vi "test Invalid Event References Leaking.vi"(8 "error in":errorcluster) -> (0 "error out":errorcluster)   [LabVIEW 2020, in "ase.test.lvlib"]
uses:
  ase.test.lvlib
  ase/ase/ase.lvclass/ase.ctl
  ase/ase/Trim Whitespace.vi
  ase/ase/Merge Call Library Errors.vi
  ase/ase/Check Shared Library Version.vi
  ase/ase/Start Call.vi/a70fc713-9ee9-4497-bede-7e71c94245f2.vi
  ase/ase/Error Invalid ASE Handle.vi
  ase/ase/Error Internal Library Implementation Error.vi
  <vilib>/Utility/file.llb/Application Directory.vi
  ase/ase/Wait on Call.vi
  <vilib>/addons/_JKI Toolkits/Caraya/classes/Assert/Assert Equal Value_Variant.vi
  ase/ase/ase.lvclass
  <vilib>/addons/_JKI Toolkits/Caraya/classes/Assert/Assert.lvclass
  <vilib>/addons/_JKI Toolkits/Caraya/classes/Test/Test.lvclass
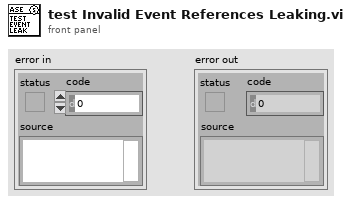
[diagram p1: front panel]
types:
  T1 = typedef "ase.lvlib/ase.lvclass/Event References.ctl" = cluster{"Standard Output":refnum<user-event>, "Standard Error":refnum<user-event>, "Did Exit":refnum<user-event>}
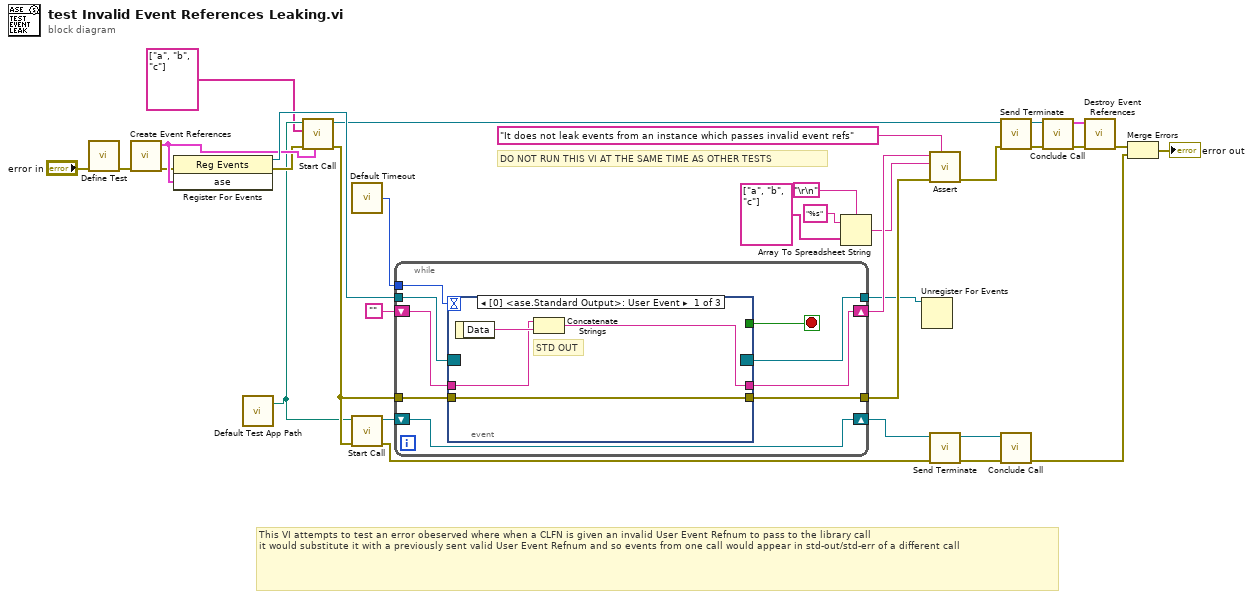
[diagram p0: block diagram]
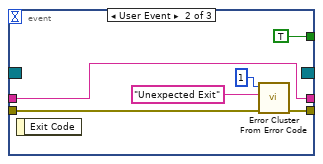
[diagram p2: hidden frame]
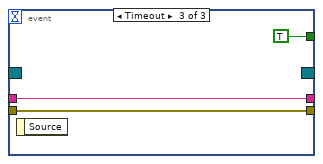
[diagram p3: hidden frame]
diagram:
  # "This VI attempts to test an error obeserved where when a CLFN is given an invalid User Event Refnum to pass to the library call\nit would substitute it with a previously sent valid User Event Refnum and so events from one call would appear in std-out/std-err of a different call"
  # "DO NOT RUN THIS VI AT THE SAME TIME AS OTHER TESTS"
  n1 = call <vilib>:"Define Test.vi"("error in (no error)"="error in") -> ("error out"=w27:errorcluster)  [unwired: 9 in, 1 out]
  n2 = call "Create Event References.vi"("error in"=w27) -> ("error out"=w25:errorcluster, "ase"=w28:T1)  [unwired: 9 in]
  n3 = register-events(error in=w25, w28) -> (reference out=w30:refnum<event-registration>, error out=w26:errorcluster)  [unwired: 1 in]
  n4 = call "Default Test App Path.vi"() -> ("Exe Path With Extention"=w3:path)  [unwired: 2 in, 1 out]
  n5 = call "Start Call.vi"("Event References"=w28, "error in"=w26, "Arguments (Default: Empty)"=string[] ["a", "b", "c"] ("Arguments"), "Executable Path"=w3) -> ("error out"=w15:errorcluster, "New ASE Handle"=w17:refnum<class "ase.lvclass">)  [unwired: 6 in]
  n6 = call "Default Timeout.vi"() -> ("Default Timeout"=w31:i32)
  n7 = call "Start Call.vi"("error in"=w15, "Executable Path"=w3) -> ("error out"=w14:errorcluster, "New ASE Handle"=w12:refnum<class "ase.lvclass">)  [unwired: 8 in]
  n8 = while {
    tunnel: w30 -> [w41]
    tunnel: [w40] -> w1
    shift-right: [w37] -> w21
    shift-left: "" ("Empty String Constant") -> [w38]
    tunnel: w31 -> [w36]
    tunnel: [w42] -> w20
    tunnel: w15 -> [w35]
    shift-right: [w34] -> w13
    shift-left: w12 -> [w34]
    stop <- w39 stop-if-true
    n9 = event shown="[0] <ase.Standard Output>: User Event" {
      selector: w41 -> [_ _ _]
      dyn-events: [_ _ _] -> w40
      timeout: w36 -> [_ _ _]
      tunnel: [w43 w50 w53] -> w42
      tunnel: [_ TRUE TRUE] -> w39
      tunnel: w38 -> [w45 w52 w54]
      tunnel: [w44 w52 w54] -> w37
      tunnel: w35 -> [w43 w47 w53]
      event User Event {
        # "STD OUT"
        n10 = event-data() -> ("Data"=w46:string)  [unwired: 1 in]
        n11 = Concatenate Strings(w45, w46) -> (w44:string)
      }
      event User Event {
        n12 = event-data() -> ()  [unwired: 1 in, 1 out]
        n13 = call <vilib>:"Error Cluster From Error Code.vi"("error in (no error)"=w47, "error message (\"\")"="Unexpected Exit" ("error message (\"\")"), "error code (0)"=1) -> ("error out"=w50:errorcluster)  [unwired: 6 in]
      }
      event Timeout {
        n14 = event-data() -> ()  [unwired: 1 in, 1 out]
      }
    }
  }
  n15 = Array To Spreadsheet String(delimiter (Tab)="\r\n", array=string[] ["a", "b", "c"] ("Arguments"), 3:"%s" ("format string")) -> (spreadsheet string=w4:string)
  n16 = Unregister For Events(event registration refnum=w1) -> ()  [unwired: 1 in, 1 out]
  n17 = call-poly <vilib>:"Assert.vi"("Label"="It does not leak events from an instance which passes invalid event refs", "error in (no error)"=w20, "Y"=w4, "X"=w21) -> ("error out"=w24:errorcluster)  [unwired: 6 in, 1 out]
  n18 = call "Send Terminate.vi"("error in"=w14, "ASE Handle"=w13) -> ("error out"=w10:errorcluster, "ASE Handle Duplicate"=w11:refnum<class "ase.lvclass">)  [unwired: 7 in, 1 out]
  n19 = call "Send Terminate.vi"("error in"=w24, "ASE Handle"=w17) -> ("error out"=w18:errorcluster, "ASE Handle Duplicate"=w16:refnum<class "ase.lvclass">)  [unwired: 7 in, 1 out]
  n20 = call "Conclude Call.vi"("error in"=w10, "ASE Handle"=w11) -> ("error out"=w8:errorcluster)  [unwired: 7 in, 2 out]
  n21 = call "Conclude Call.vi"("error in"=w18, "ASE Handle"=w16) -> ("error out"=w23:errorcluster, "Event References"=w19:T1)  [unwired: 7 in, 1 out]
  n22 = call "Destroy Event References.vi"("error in"=w23, "Event References"=w19) -> ("error out"=w22:errorcluster)  [unwired: 9 in]
  n23 = Merge Errors(w22, w8) -> (→"error out":errorcluster)
